vi "Table Exists.vi"(8 "error in (no error)":errorcluster, 10 "table":string, 11 "SQLite3LV Cursor in":refnum<class "cursor.lvclass">) -> (0 "error out":errorcluster, 2 "exists?":bool, 3 "SQLite3LV Cursor out":refnum<class "cursor.lvclass">)   [LabVIEW 2014, in "SQLite3LV.lvlib" / "cursor.lvclass"]
doc: "A utility function that checks if the specified table exists."
uses:
  cursor.lvclass
  property binding/bind text.vi
  property binding/column I32.vi
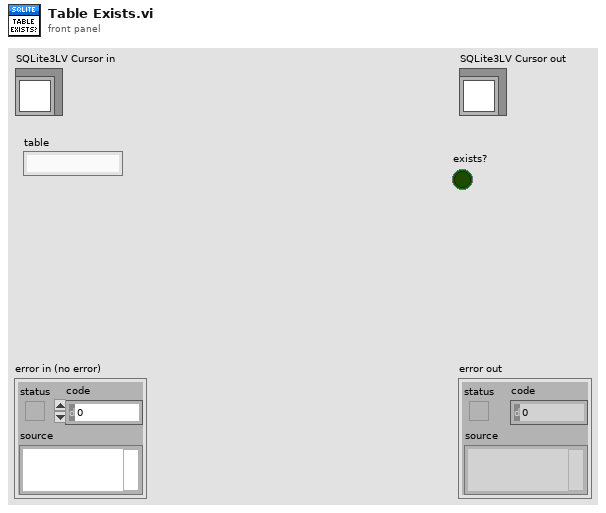
[diagram p1: front panel]
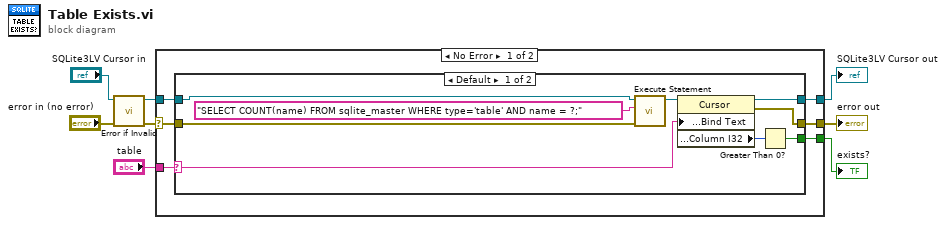
[diagram p0: block diagram]
diagram:
  n1 = call "Error if Invalid.vi"("error in (no error)"="error in (no error)", "SQLite3LV Cursor in"="SQLite3LV Cursor in") -> ("error out"=w2:errorcluster, "SQLite3LV Cursor out"=w3:refnum<class "cursor.lvclass">)  [unwired: 8 in]
  n2 = case shown="No Error" w2 {
    selector: w2 -> [w14 w27]
    tunnel: [w13 w27] -> w8
    tunnel: [w12 w26] -> w7
    tunnel: w3 -> [w10 w26]
    tunnel: "table" -> [w11 _]
    tunnel: [w9 _] -> w1
    frame No Error {
      n3 = case shown="Default" w11 {
        selector: w11 -> [w21 _]
        tunnel: w14 -> [w23 w25]
        tunnel: [w16 w25] -> w13
        tunnel: [w15 w24] -> w12
        tunnel: w10 -> [w20 w24]
        tunnel: [w17 _] -> w9
        frame Default {
          n4 = call "Execute Statement.vi"("error in (no error)"=w23, "SQL statement"="SELECT COUNT(name) FROM sqlite_master WHERE type='table' AND name = ?;" ("statement"), "SQLite3LV Cursor in"=w20) -> ("SQLite3LV Cursor out"=w19:refnum<class "cursor.lvclass">)  [unwired: 7 in, 1 out]
          n5 = property class="Cursor"(reference=w19, "property binding:Bind Text"=w21) -> (reference out=w15:refnum<class "cursor.lvclass">, error out=w16:errorcluster, "property binding:Column I32"=w18:i32)  [unwired: 1 in]
          n6 = Greater Than 0?(x=w18) -> (x > 0?=w17:bool)
        }
        frame "" {
        }
      }
    }
    frame Error {
    }
  }
  "error out" <- w8
  "SQLite3LV Cursor out" <- w7
  "exists?" <- w1
